vi "Box Colour Detection SubVI.vi"(0 "Image In":T2, 1 "Error In":errorcluster) -> (2 "Classes (Color Classification 1)":string[](array[string]), 3 "Colour output boolean cluster":T1, 4 "Error out":errorcluster)   [LabVIEW 2018]
uses:
  <vilib>/vision/Classification.llb/IMAQ Classifier Session.ctl
  <vilib>/vision/Image Controls.llb/IMAQ Image.ctl
panel:
  out "?":bool
  out "VI loop iteration":i32
  out "White":bool
  out "Green":bool
  out "Yellow":bool
  out "Blue":bool
  out "Black":bool
  out "Red":bool
  out "Classifier Session (Color Classification 1)":T3
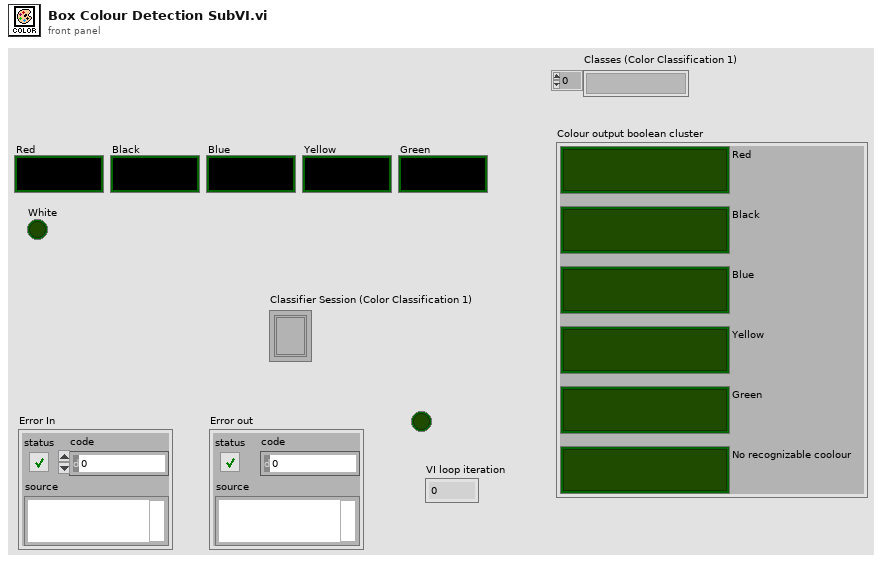
[diagram p1: front panel]
types:
  T1 = cluster{"Red":bool, "Black":bool, "Blue":bool, "Yellow":bool, "Green":bool, "No recognizable coolour":bool}
  T2 = typedef "IMAQ Image.ctl" = refnum<image>
  T3 = typedef "IMAQ Classifier Session.ctl" = refnum<k1>
  T4 = cluster{"Classes (Color Classification 1)[0]":string, "Classes (Color Classification 1)[1]":string, "Classes (Color Classification 1)[2]":string, "Classes (Color Classification 1)[3]":string, "Classes (Color Classification 1)[4]":string, "Classes (Color Classification 1)[5]":string, "Classes (Color Classification 1)[6]":string, "Classes (Color Classification 1)[7]":string, "Classes (Color Classification 1)[8]":string}
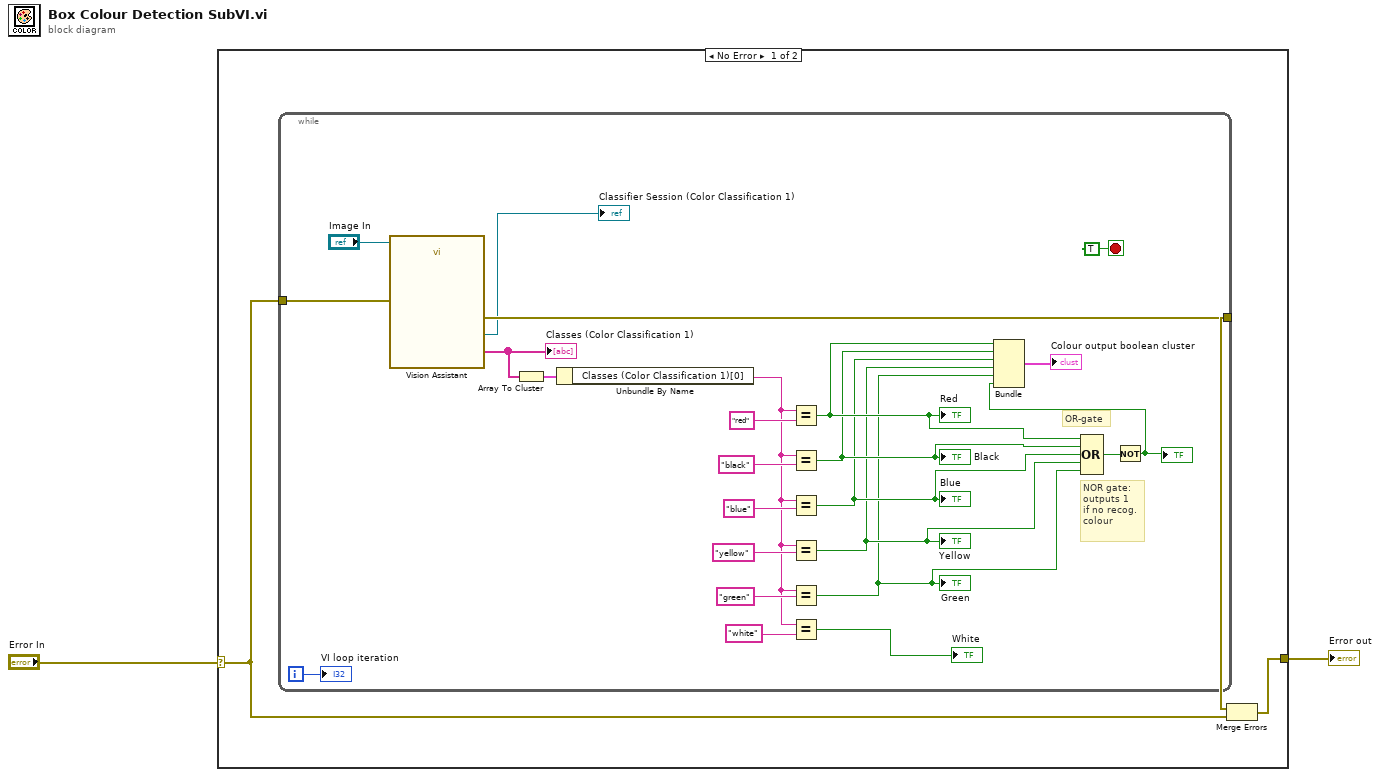
[diagram p0: block diagram]
diagram:
  n1 = case shown="No Error" "Error In" {
    selector: "Error In" -> [w4 w30]
    tunnel: [w5 w30] -> w1
    frame No Error {
      n2 = while {
        tunnel: w4 -> [w26]
        tunnel: [w29] -> w3
        i -> [w14]
        stop <- TRUE ("Stop (F)") stop-if-true
        # "NOR gate:\noutputs 1 \nif no recog.\ncolour"
        # "OR-gate"
        n3 = call "Vision Assistant"("Image In"="Image In", "error in"=w26) -> ("Classifier Session (Color Classification 1)"=→"Classifier Session (Color Classification 1)":T3, "Classes (Color Classification 1)"=w25:string[], "error out"=w29:errorcluster)  [unwired: 22 in, 1 out]
        "Classes (Color Classification 1)" <- w25
        n4 = Array To Cluster(array=w25) -> (cluster=w24:T4)
        n5 = Unbundle By Name(w24) -> ("Classes (Color Classification 1)[0]"=w17:string)
        n6 = Equal?(x=w17, y="red") -> (x = y?=w12:bool)
        "Red" <- w12
        n7 = Equal?(x=w17, y="black") -> (x = y?=w11:bool)
        "Black" <- w11
        n8 = Equal?(x=w17, y="blue") -> (x = y?=w10:bool)
        "Blue" <- w10
        n9 = Equal?(x=w17, y="yellow") -> (x = y?=w9:bool)
        "Yellow" <- w9
        n10 = Equal?(x=w17, y="green") -> (x = y?=w8:bool)
        "Green" <- w8
        n11 = Equal?(x=w17, y="white") -> (x = y?=→"White":bool)
        n12 = Compound Arithmetic op=OR(w12, w11, w10, w9, w8) -> (w7:bool)
        n13 = Not(x=w7) -> (.not. x?=w6:bool)
        "?" <- w6
        n14 = Bundle(w12, w11, w10, w9, w8, w6) -> (→"Colour output boolean cluster":cluster{bool, bool, bool, bool, bool, bool})  [unwired: 1 in]
        "VI loop iteration" <- w14
      }
      n15 = Merge Errors(w3, w4) -> (w5:errorcluster)
    }
    frame Error {
    }
  }
  "Error out" <- w1
